vi "interlock v1.vi"() -> ()   [LabVIEW 2015]
panel:
  out "Turbo Status Array":bool[](array[boolean])
  in  "Task to Check Array":refnum<k21>[](array[refnum])
  in  "Test Array":dbl[](array[numeric])
  in  "Turbo Test Array":bool[](array[boolean])
  in  "Manual Test Array":bool[](array[boolean])
  in  "120V Test Array":bool[](array[boolean])
  in  "GV Test Array":bool[](array[boolean])
  out "Manual Control Array":bool[](array[boolean])
  out "120V Relay Signals":refnum<k21>[](array[refnum])
  out "P2L0 in Array":refnum<k21>[](array[refnum])
  out "previous state":bool[](array[boolean])
  out "current state array":bool[](array[boolean])
  out "gv open array":bool[](array[boolean])
  out "gv close array":bool[](array[boolean])
  out "is safe array":bool[](array[boolean])
  out "P0L0 out Array":refnum<k21>[](array[refnum])
  out "P0L16 out Array":refnum<k21>[](array[refnum])
  out "P0L8 in Array":refnum<k21>[](array[refnum])
  in  "Tab Control":enum32{"Page 1"}(tab)
  out "element 5":bool
  out "element 4":bool
  out "Error Indicator":bool
  out "Turbo 1 Status":bool
  out "Turbo 2 Status":bool
  in  "Warnings Cluster":T1
  in  "Turbo Test 1":bool
  in  "Turbo Test 2":bool
  in  "Turbo Test 3":bool
  in  "OK Button":bool
  out "ERROR A":errorcluster
  in  "Beamline 2 Test":dbl
  in  "Beamline 3 Test":dbl
  in  "LEIL Test":dbl
  in  "Turbo 1 Test":dbl
  in  "Turbo 2 Test":dbl
  in  "Turbo 3 Test":dbl
  in  "Post Leil Test":dbl
  in  "Micro Ion Test":dbl
  in  "Beamline 1 Test":dbl
  in  "120V Relay Test 1":bool
  in  "120V Relay Test  2":bool
  in  "120V Relay Test  3":bool
  in  "120V Relay Test  4":bool
  in  "120V Relay Test  5":bool
  in  "120V Relay Test  6":bool
  in  "120V Relay Test  7":bool
  in  "120V Relay Test  8":bool
  in  "Manual Test 1":bool
  in  "Manual Test 2":bool
  in  "Manual Test 3":bool
  in  "Manual Test 4":bool
  in  "Manual Test 5":bool
  in  "Manual Test 6":bool
  in  "Manual Test 7":bool
  in  "Manual Test 8":bool
  in  "GV TEST 1":bool
  in  "GV TEST 2":bool
  in  "GV TEST 3":bool
  in  "GV TEST 4":bool
  in  "GV TEST 5":bool
  in  "GV TEST 6":bool
  in  "GV TEST 7":bool
  in  "GV TEST 8":bool
  in  "TEST MODE":bool
  in  "Pressure Trest Mode":bool
  in  "GV Test Mode":bool
  in  "120 V Status Test Mode":bool
  in  "Turbo Status Test Mode":bool
  in  "Manual Test Mode":bool
  out "SV 1":bool
  out "SV2":bool
  out "SV3":bool
  in  "stop":bool
  out "High Voltage Status":bool
  out "Turbo 2":dbl format="%#_2e"
  in  "OK Button 9":bool
  in  "OK Button 8":bool
  in  "OK Button 7":bool
  in  "OK Button 6":bool
  in  "OK Button 5":bool
  in  "OK Button 4":bool
  in  "OK Button 3":bool
  in  "OK Button 2":bool
  out "GV 8 Status":bool
  out "Gv 7 Status":bool
  out "GV 6 Status":bool
  out "GV 5 Status":bool
  out "GV 4 Status":bool
  out "GV 2 Status":bool
  out "Turbo 2 Backing":bool
  out "Mode 1":bool
  out "Mode 2":bool
  out "Mode 3":bool
  out "Mode 4":bool
  out "Mode 5":bool
  out "GV 1 Status":bool
  out "GV 2 Status":bool
  out "GV 3 Status":bool
  out "GV 4 Status":bool
  out "GV 5 Status":bool
  in  "GV 1":bool
  in  "GV 2":bool
  in  "GV 3":bool
  in  "GV 4":bool
  in  "GV 5":bool
  out "Mode 6":bool
  in  "GV 6":bool
  out "GV 6 Status":bool
  out "Mode 7":bool
  in  "GV 7":bool
  out "GV 7 Status":bool
  out "Mode 8":bool
  in  "GV 8":bool
  out "GV 8 Status":bool
  out "120 V 4 Status":bool
  out "120 V 3 Status":bool
  out "120 V 2 Status":bool
  out "GV 3 Status":bool
  out "GV 1 Status":bool
  out "Cryo 2 Pressure":bool
  out "Cryo 2 Status":bool
  out "Turbo 3 Status":bool
  out "RGA 2 Status":bool
  out "RGA 1 Status":bool
  out "Cryo 1 Status":bool
  out "Cryo 1 Pressure":bool
  out "Beamline 2":dbl format="%#_2e"
  out "Source Electronics Status":bool
  out "Beamline 3":dbl format="%#_2e"
  out "Turbo 1":dbl format="%#_2e"
  out "120 V 1 Status":bool
  out "Micro Ion":dbl format="%#_2e"
  out "Beamline 1":dbl format="%#_2e"
  out "LEIL":dbl format="%#_2e"
  out "Turbo 3":dbl format="%#_2e"
  out "Pos Leil":dbl format="%#_2e"
  out "Post LEIL Pressure":bool
  out "Cryo 2":bool
  out "Beamline 3":bool
  out "Beamline 2 S":bool
  out "LEIL Pressure":bool
  out "Beamline 1 S":bool
  out "Cryo 1":bool
  out "Turbo 1 Backing":bool
  out "Turbo 3 Backing":bool
  out "element":bool
  out "element 2":bool
  out "element 3":bool
  # "RGA 2"
  # "Stutus"
  # "Turbo 1"
  # "Turbo 2"
  # "RGA 1"
  # "Spinning \nStatus"
  # "Turbo 3"
  # "Spinning \nStatus"
  # "Stutus"
  # "Spinning \nStatus"
  # "1\n            2\n            3 \n           4 \n           5  \n          6 \n           7  \n          8"
  # "GV 7"
  # "GV 4"
  # "GV 1"
  # "GV 6"
  # "GV 2"
  # "GV 8"
  # "GV 5"
  # "PSU"
  # "GV 3"
  # "8              7             6             5              4              3              2              1"
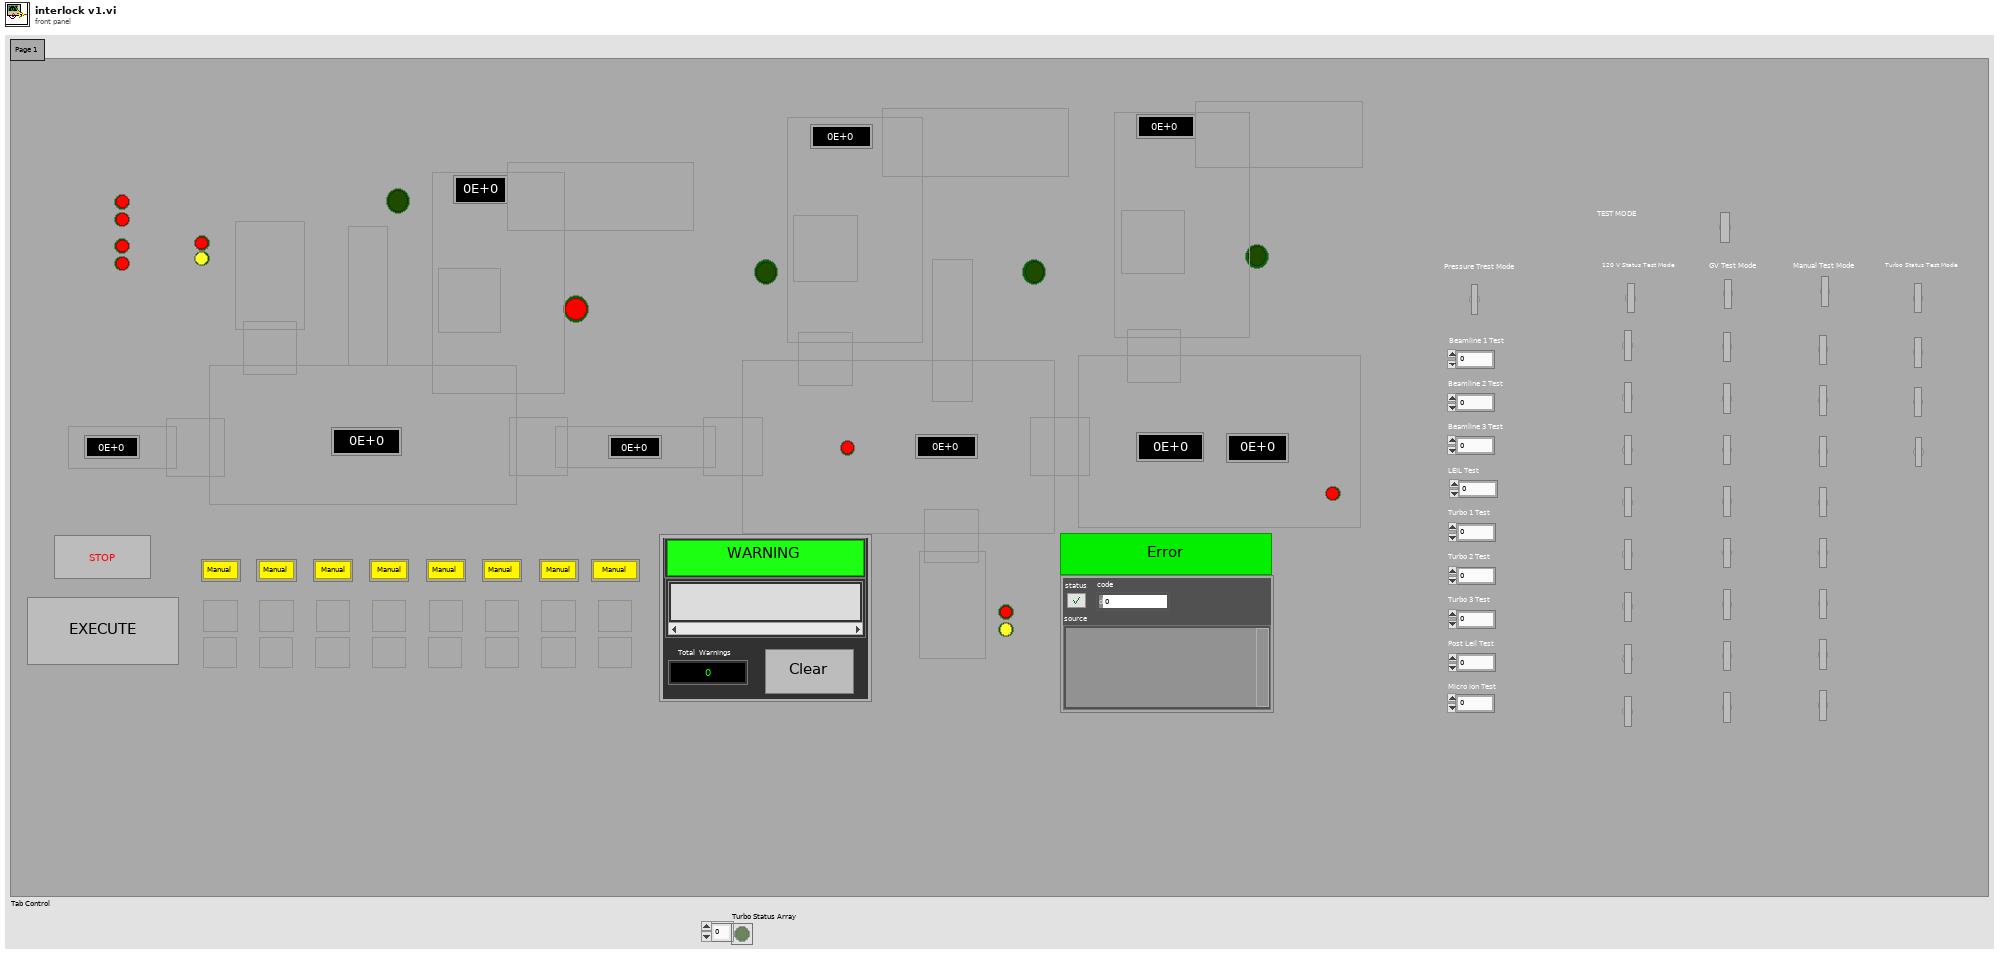
[diagram p1: front panel]
types:
  T1 = cluster{"Warning Array Out":string[], "Clear":bool, "Existing Warnings":i32[], "Num Warning Queue":i32[], "Total  Warnings":i32, "OK Button":bool, "Warning Indicator":bool}
  T2 = enum8{"Enabled", "Disabled", "Disabled and Grayed Out"}
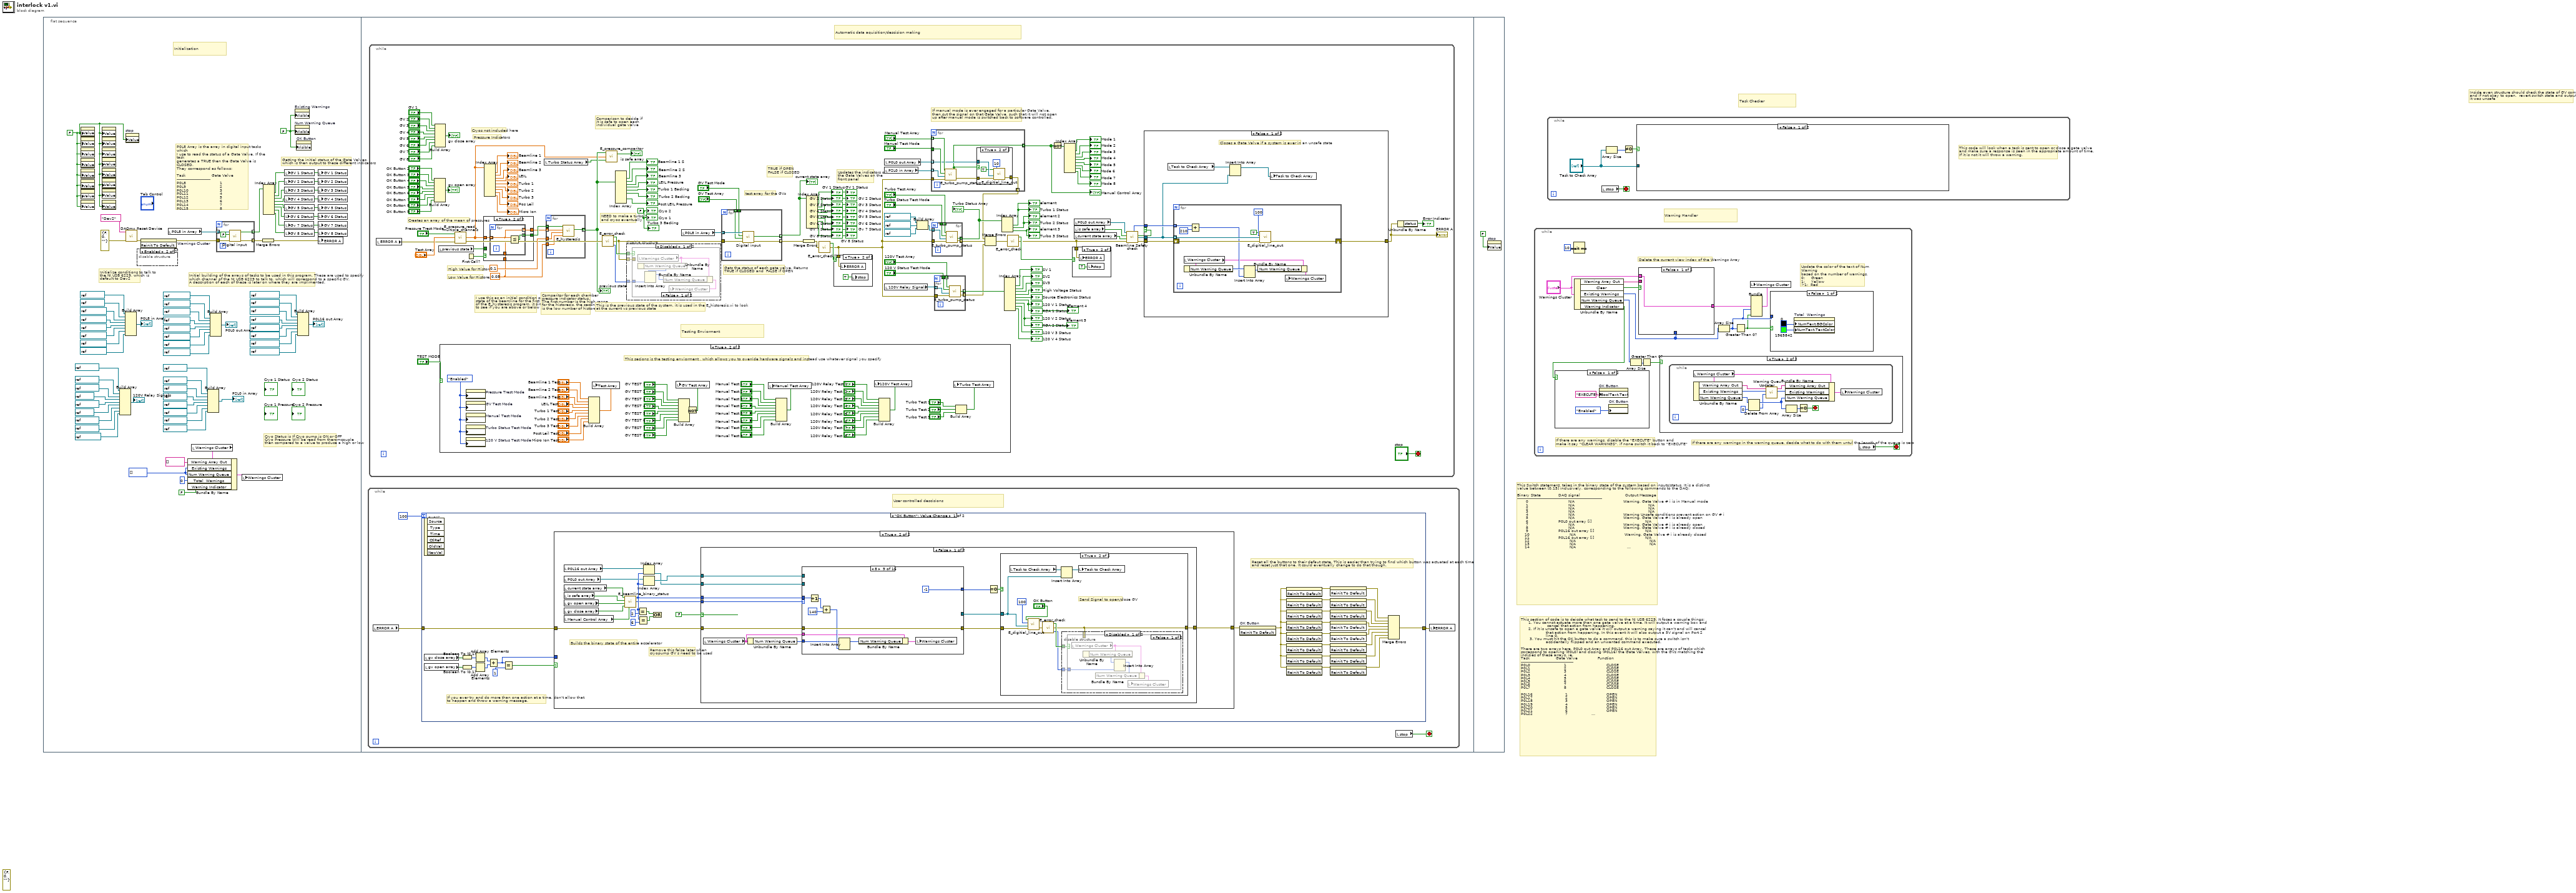
[diagram p0: block diagram]
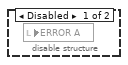
[diagram p2: hidden frame]
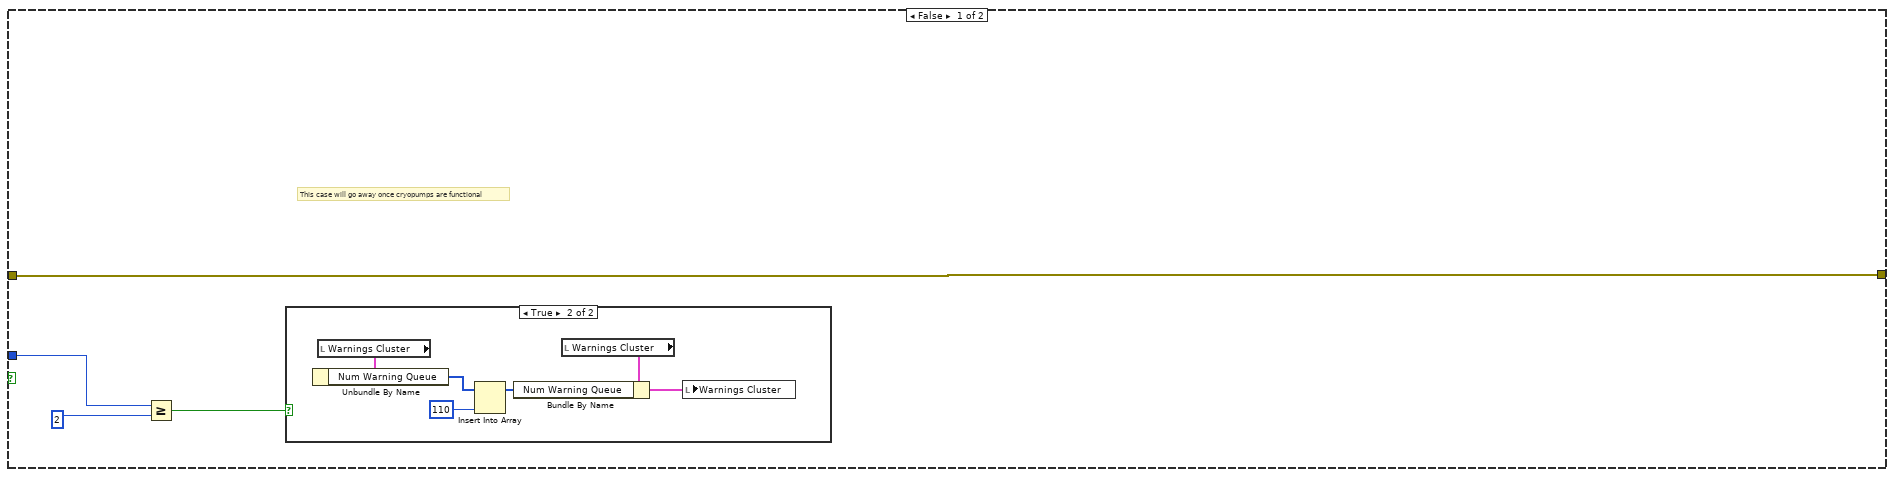
[diagram p3: hidden frame]
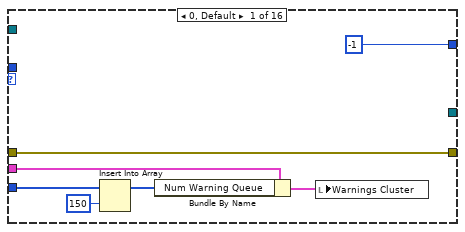
[diagram p5: hidden frame]
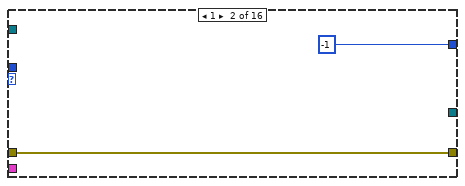
[diagram p6: hidden frame]
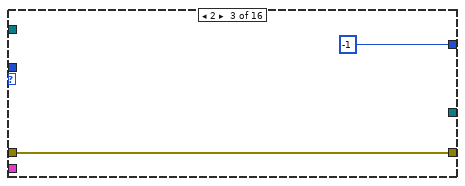
[diagram p7: hidden frame]
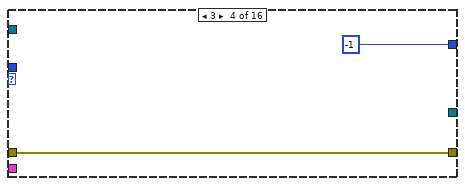
[diagram p8: hidden frame]
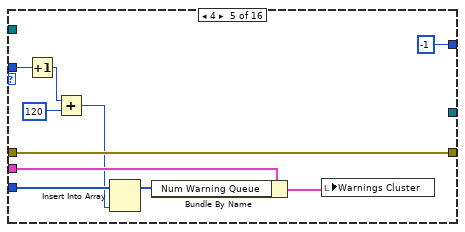
[diagram p9: hidden frame]
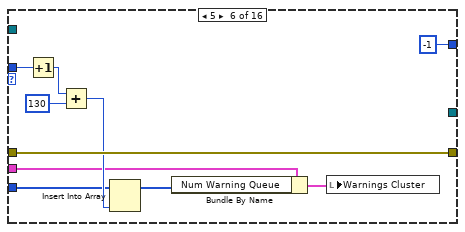
[diagram p10: hidden frame]
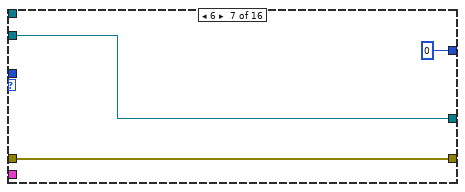
[diagram p11: hidden frame]
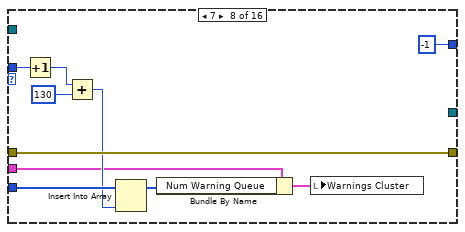
[diagram p12: hidden frame]
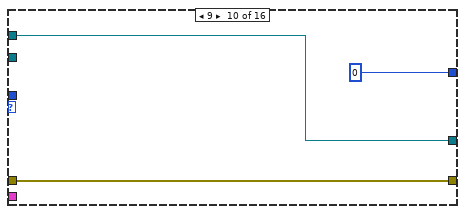
[diagram p13: hidden frame]
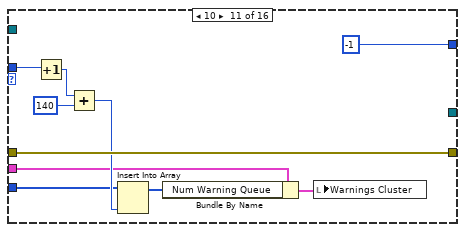
[diagram p14: hidden frame]
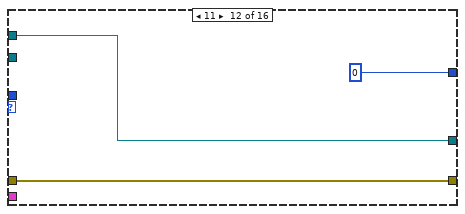
[diagram p15: hidden frame]
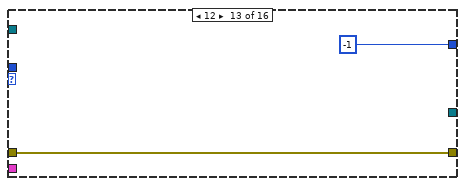
[diagram p16: hidden frame]
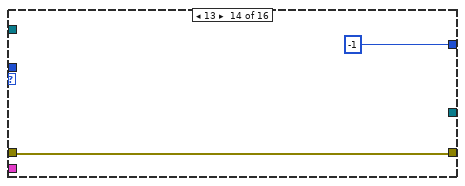
[diagram p17: hidden frame]
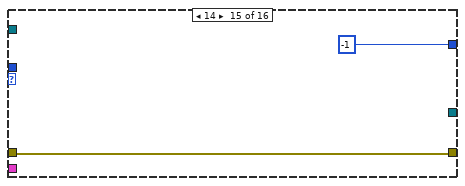
[diagram p18: hidden frame]
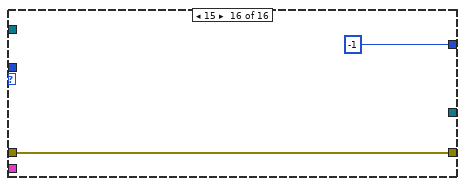
[diagram p19: hidden frame]
diagram:
  (unwired) errorcluster {"status"=FALSE, "code"=0, "source"=""} ("error out")
  # "Task Checker"
  # "Warning Handler"
  # "This Switch statement  takes in the binary state of the system based on inputs/status. It is a distinct\nvalue between [0,15] inclusively, corresponding to the following commands to the DAQ:\n\nBinary State              DAQ signal                                    Output Message\n--------------------------------------------------------------------  \n       0                                N/A                                       Warning, Gate Valve # i is in Manual mode\n       1                                N/A                                                           N/A\n       2                                N/A                                                           N/A\n       3                                N/A                                                           N/A\n       4                                N/A                                       Warning Unsafe conditions prevent action on GV # i\n       5                                N/A                                       Warning, Gate Valve # i is already open\n       6                        P0L0 out array [i]                                           N/A\n       7                                N/A                                       Warning, Gate Valve # i is already open\n       8                                N/A                                       Warning, Gate Valve # i is already closed\n       9                        P0L16 out array [i]                                         N/A\n      10                                N/A                                       Warning, Gate Valve # i is already closed\n      11                       P0L16 out array [i]                                         N/A\n      12                                N/A                                                           N/A\n      13                                N/A                                                           N/A\n      14                                N/A                                                           N/A\n      15                                N/A                                                           N/A\n\nwhere i is the index of the array which corresponds to the Gate valve number.  A description of \nwhat each of these signals does can be found above. \n\nAs a note, the states of between [1,3] inclusively and [12,15] are disallowed states based on the\narchitecture of how the numbers are built and constraints on not being able to have 0 or more than \n1 button hit at a time. I'll consider removing these from the switch statement."
  # "This section of code is to deicde what task to send to the NI USB 6229. It foces a couple things:\n      1. You cannot actuate more than one gate valve at a time. It will output a warning box and \n                     cancel that action from happening.\n      2. If it is unsafe to open a gate valve it will output a warning saying it can't and will cancel \n                    that action from happening. In this event it will also output a 5V signal on Port 2 \n                    line 0.\n       3. You must hit the OK button to do a command, this is to make sure a switch isn't\n                    accidentally flipped and an unwanted command executed.\n\nThere are two arrays here, P0L0 out Array and P0L16 out Array. These are arrays of tasks which \ncorrespond to opening (P0L0) and closing (P0L16) the Gate Valves, with the GVs matching the \nindicies of these arrays. ie. \nTask                     Gate Valve                Function\n------------------------------------------\nP0L0                           1                                CLOSE\nP0L1                           2                                CLOSE\nP0L2                           3                                CLOSE\nP0L3                           4                                CLOSE\nP0L4                           5                                CLOSE\nP0L5                           6                                CLOSE\nP0L6                           7                                CLOSE\nP0L7                           8                                CLOSE\n  \nP0L16                          1                               OPEN\nP0L17                          2                               OPEN\nP0L18                          3                               OPEN\nP0L19                          4                               OPEN\nP0L20                          5                               OPEN\nP0L21                          6                               OPEN\nP0L22                          7                               OPEN\nP0L23                          8                               OPEN"
  # "Inside even structure should check the state of GV comparison array,\nand if not okay to open,  revert switch state and output a message saying\nit was unsafe"
  n1 = flat-sequence {
    frame #0 {
      w2 = FALSE ("GV 1")
      w9 = i32[] [] ("Existing Warnings")
      w13 = FALSE ("Visible")
      # "Initialization"
      # "Cryo Status is If Cryo pump is ON or OFF\nCryo Pressure Will be read from theromcouple \nthen compared to a value to produce a high or low"
      # "Initialize conditions to talk to\nthe NI USB 6229, which is \ndefault to Dev2"
      # "P0L8 Array is the array in digital input tasks which \nI use to read the status of a Gate Valve. If the task\ngenerates a TRUE then the Gate Valve is CLOSED.\nThey corrrespond as follows:\n\nTask                     Gate Valve     \n---------------------------\nP0L8                           1                                \nP0L9                           2                                \nP0L10                         3                               \nP0L11                         4                                \nP0L12                         5                                \nP0L13                         6                                \nP0L14                         7                               \nP0L15                         8"
      # "Getting the initial status of the Gate Valves,\nwhich is then output to these different indicators"
      # "Initial building of the arrays of tasks to be used in this program. These are used to specify\nwhich channel of the NI USB 6229 to talk to, which will correspond to a specific GV. \nA description of each of these is later on where they are implimented."
      n2 = property on="GV 1" class="Bool (strict)"("Value"=w2) -> ()  [unwired: 2 in, 2 out]
      n3 = property on="GV 2" class="Bool (strict)"("Value"=w2) -> ()  [unwired: 2 in, 2 out]
      n4 = property on="GV 3" class="Bool (strict)"("Value"=w2) -> ()  [unwired: 2 in, 2 out]
      n5 = property on="GV 4" class="Bool (strict)"("Value"=w2) -> ()  [unwired: 2 in, 2 out]
      n6 = property on="GV 5" class="Bool (strict)"("Value"=w2) -> ()  [unwired: 2 in, 2 out]
      n7 = property on="GV 6" class="Bool (strict)"("Value"=w2) -> ()  [unwired: 2 in, 2 out]
      n8 = property on="GV 7" class="Bool (strict)"("Value"=w2) -> ()  [unwired: 2 in, 2 out]
      n9 = property on="GV 8" class="Bool (strict)"("Value"=w2) -> ()  [unwired: 2 in, 2 out]
      n10 = property on="OK Button 2" class="Bool (strict)"("Value"=w2) -> ()  [unwired: 2 in, 2 out]
      n11 = property on="OK Button 3" class="Bool (strict)"("Value"=w2) -> ()  [unwired: 2 in, 2 out]
      n12 = property on="OK Button 4" class="Bool (strict)"("Value"=w2) -> ()  [unwired: 2 in, 2 out]
      n13 = property on="OK Button 5" class="Bool (strict)"("Value"=w2) -> ()  [unwired: 2 in, 2 out]
      n14 = property on="OK Button 6" class="Bool (strict)"("Value"=w2) -> ()  [unwired: 2 in, 2 out]
      n15 = property on="OK Button 7" class="Bool (strict)"("Value"=w2) -> ()  [unwired: 2 in, 2 out]
      n16 = property on="OK Button 8" class="Bool (strict)"("Value"=w2) -> ()  [unwired: 2 in, 2 out]
      n17 = property on="OK Button 9" class="Bool (strict)"("Value"=w2) -> ()  [unwired: 2 in, 2 out]
      n18 = Build Array(refnum<k21> "P2L0 in" ("task/channels in"), refnum<k21> "P2L1 in" ("task/channels in"), refnum<k21> "P2L2 in" ("task/channels in"), refnum<k21> "P2L3" ("task/channels in"), refnum<k21> "P2L4 in" ("task/channels in"), refnum<k21> "P2L5" ("task/channels in"), refnum<k21> "P2L6 in" ("task/channels in"), refnum<k21> "P2L7 in" ("element"), refnum<k21> "P0L24 in" ("element")) -> (→"120V Relay Signals":refnum<k21>[])
      n19 = Build Array(refnum<k21> "P0L8 in" ("task/channels in"), refnum<k21> "P0L9 in" ("task/channels in"), refnum<k21> "P0L10 in" ("task/channels in"), refnum<k21> "P0L11 in" ("task/channels in"), refnum<k21> "P0L12 in" ("task/channels in"), refnum<k21> "P0L13 in" ("task/channels in"), refnum<k21> "P0L14 in" ("task/channels in"), refnum<k21> "P0L15 in" ("element")) -> (→"P0L8 in Array":refnum<k21>[])
      n20 = property on="stop" class="Bool (strict)"("Value"=w2) -> ()  [unwired: 2 in, 2 out]
      n21 = call <vilib>:"DAQmx Reset Device.vi"("device in"=tag "Dev2", "error in"=errorcluster {"status"=FALSE, "code"=0, "source"=""} ("error out")) -> ("error out"=w11:errorcluster)  [unwired: 13 in]
      n22 = disable-structure shown="Enabled" {
        frame Disabled {
          n23 = local read "ERROR A"() -> ()  [unwired: 1 in]
        }
        frame Enabled {
        }
      }
      n24 = invoke on="Warnings Cluster" class="Clust (strict)" method="Reinit To Default"(error in=w11) -> (error out=w12:errorcluster)  [unwired: 2 in, 2 out]
      n25 = local read "P0L8 in Array"() -> (w51:refnum<k21>[])
      n26 = local read "Warnings Cluster"() -> (w10:T1)
      n27 = Bundle By Name(cluster=w10, "Warning Array Out"=string[] [], "Existing Warnings"=w9, "Num Warning Queue"=w9, "Total  Warnings"=0, "Warning Indicator"=FALSE) -> (w5:T1)
      n28 = Build Array(refnum<k21> "P1L0 in" ("task/channels in"), refnum<k21> "P1L1 in" ("task/channels in"), refnum<k21> "P1L2 in" ("task/channels in"), refnum<k21> "P1L3 in" ("task/channels in"), refnum<k21> "P1L4 in" ("task/channels in"), refnum<k21> "P1L5 in" ("task/channels in"), refnum<k21> "P1L6 in" ("task/channels in"), refnum<k21> "P1L7 in" ("element")) -> (→"P2L0 in Array":refnum<k21>[])
      n29 = Build Array(refnum<k21> "P0L0 out" ("task/channels in"), refnum<k21> "P0L1 out" ("task/channels in"), refnum<k21> "P0L2 out" ("task/channels in"), refnum<k21> "P0L3 out" ("task/channels in"), refnum<k21> "P0L4 out" ("task/channels in"), refnum<k21> "P0L5 out" ("task/channels in"), refnum<k21> "P0L6 out" ("task/channels in"), refnum<k21> "P0L7 out" ("element")) -> (→"P0L0 out Array":refnum<k21>[])
      n30 = for {
        tunnel: w12 -> [w75]
        tunnel: [w74] -> w69 mode=indexing
        tunnel: w51 -> [w73] mode=indexing
        tunnel: [w72] -> w1 mode=indexing
        n31 = call "Digital input.vi"("error in"=w75, "test"=FALSE, "task/channels in"=w73) -> ("error out"=w74:errorcluster, "element 2"=w72:bool)  [unwired: 7 in]
      }
      n32 = local write "Warnings Cluster"(w5) -> ()
      n33 = Merge Errors(w69) -> (w3:errorcluster)
      n34 = Index Array(array=w1) -> (element #1=w68:bool, element #2=w67:bool, element #3=w66:bool, element #4=w65:bool, element #5=w64:bool, element #6=w63:bool, element #7=w62:bool, element #8=w61:bool)  [unwired: 8 in]
      n35 = local write "GV 6 Status"(w63) -> ()
      n36 = local write "GV 1 Status"(w68) -> ()
      n37 = local write "GV 2 Status"(w67) -> ()
      n38 = local write "GV 3 Status"(w66) -> ()
      n39 = local write "GV 4 Status"(w65) -> ()
      n40 = local write "GV 5 Status"(w64) -> ()
      n41 = local write "Gv 7 Status"(w62) -> ()
      n42 = local write "GV 8 Status"(w61) -> ()
      n43 = property on="Existing Warnings" class="Arr (strict)"("Visible"=w13) -> ()  [unwired: 2 in, 2 out]
      n44 = property on="Num Warning Queue" class="Arr (strict)"("Visible"=w13) -> ()  [unwired: 2 in, 2 out]
      n45 = property on="OK Button" class="Bool (strict)"("Visible"=w13) -> ()  [unwired: 2 in, 2 out]
      n46 = Build Array(refnum<k21> "P0L16 out" ("task/channels in"), refnum<k21> "P0L17 out" ("task/channels in"), refnum<k21> "P0L18 out" ("task/channels in"), refnum<k21> "P0L19 out" ("task/channels in"), refnum<k21> "P0L20 out" ("task/channels in"), refnum<k21> "P0L21 out" ("task/channels in"), refnum<k21> "P0L22 out" ("task/channels in"), refnum<k21> "P0L23 out" ("element")) -> (→"P0L16 out Array":refnum<k21>[])
      n47 = local write "GV 1 Status"(w68) -> ()
      n48 = local write "GV 2 Status"(w67) -> ()
      n49 = local write "GV 3 Status"(w66) -> ()
      n50 = local write "GV 4 Status"(w65) -> ()
      n51 = local write "GV 5 Status"(w64) -> ()
      n52 = local write "GV 6 Status"(w63) -> ()
      n53 = local write "GV 7 Status"(w62) -> ()
      n54 = local write "GV 8 Status"(w61) -> ()
      n55 = local write "ERROR A"(w3) -> ()
    }
    frame #1 {
      # "Automatic data aquisition/descision making"
      n56 = while {
        stop <- w79 stop-if-true
        # "User controlled descisions"
        n57 = local read "ERROR A"() -> (w76:errorcluster)
        n58 = event shown="[0] \"OK Button\": Value Change" {
          selector: _ -> [_ _]
          dyn-events: _ -> [_ _]
          timeout: 100 -> [_ _]
          tunnel: [w83 w256] -> w77
          tunnel: w76 -> [w80 w256]
          event "OK Button": Value Change {
            # "Reset all the buttons to their defaut state. This is easier than trying to find which button was actuated at each time\nand reset just that one. It could eventually change to do that though."
            # "If you ever try and do more than one action at a time, don't allow that \nto happen and throw a warning message."
            n59 = event-data() -> ()  [unwired: 1 in, 6 out]
            n60 = local read "gv close array"() -> (w107:bool[])
            n61 = local read "gv open array"() -> (w108:bool[])
            n62 = Boolean To (0,1)(Boolean=w107) -> (0, 1=w105:i16[])
            n63 = Boolean To (0,1)(Boolean=w108) -> (0, 1=w106:i16[])
            n64 = Add Array Elements(numeric array=w105) -> (sum=w103:i16)
            n65 = Add Array Elements(numeric array=w106) -> (sum=w104:i16)
            n66 = Add(x=w103, y=w104) -> (x+y=w100:i16)
            n67 = Equal?(x=w100, y=i16 1) -> (x = y?=w101:bool)
            n68 = case shown="True" w101 {
              tunnel: w100 -> [w110 _]
              tunnel: [w109 w119] -> w82
              tunnel: w80 -> [w109 w120]
              frame False {
                # "This case will go away once cryopumps are functional"
                n69 = Greater Or Equal?(x=w110, y=i16 2) -> (x >= y?=w111:bool)
                n70 = case shown="True" w111 {
                  frame False {
                  }
                  frame True {
                    n71 = local read "Warnings Cluster"() -> (w114:T1)
                    n72 = Unbundle By Name(w114) -> ("Num Warning Queue"=w118:i32[])
                    n73 = Insert Into Array(array=w118, new element=110) -> (w117:i32[])  [unwired: 1 in]
                    n74 = local read "Warnings Cluster"() -> (w113:T1)
                    n75 = Bundle By Name(cluster=w113, "Num Warning Queue"=w117) -> (w116:T1)
                    n76 = local write "Warnings Cluster"(w116) -> ()
                  }
                }
              }
              frame True {
                # "Builds the binary state of the entire accelerator"
                # "Remove this false later when \ncryopump GV s need to be used"
                n77 = local read "P0L16 out Array"() -> (w127:refnum<k21>[])
                n78 = local read "P0L0 out Array"() -> (w126:refnum<k21>[])
                n79 = local read "current state array"() -> (w125:bool[])
                n80 = local read "is safe array"() -> (w124:bool[])
                n81 = local read "gv open array"() -> (w123:bool[])
                n82 = local read "gv close array"() -> (w122:bool[])
                n83 = local read "Manual Control Array"() -> (w121:bool[])
                n84 = call "E_beamline_binary_status.vi"("Current State Array"=w125, "is safe array"=w124, "gv open aray"=w123, "manual mode array"=w121, "gv closed array"=w122) -> ("index"=w130:i32, "binary state"=w129:i16)  [unwired: 2 in]
                n85 = Equal?(x=w130, y=2) -> (x = y?=w136:bool)
                n86 = Equal?(x=w130, y=6) -> (x = y?=w135:bool)
                n87 = Index Array(array=w127, index=w130) -> (element=w131:refnum<k21>)
                n88 = Index Array(array=w126, index=w130) -> (element=w132:refnum<k21>)
                n89 = Or(x=w136, y=w135) -> ()  [unwired: 1 out]
                n90 = case shown="False" FALSE {
                  tunnel: [w148 w255] -> w119
                  tunnel: w120 -> [w147 w255]
                  tunnel: w132 -> [w146 _]
                  tunnel: w131 -> [w145 _]
                  tunnel: w129 -> [w140 _]
                  tunnel: w130 -> [w139 _]
                  frame False {
                    n91 = local read "Warnings Cluster"() -> (w137:T1)
                    n92 = Unbundle By Name(w137) -> ("Num Warning Queue"=w138:i32[])
                    n93 = case shown="8" w140 {
                      tunnel: [_ _ _ _ _ _ w184 _ _ w207 _ w220 _ _ _ _] -> w144
                      tunnel: w146 -> [_ _ _ _ _ _ _ _ _ w207 _ w220 _ _ _ _]
                      tunnel: w145 -> [_ _ _ _ _ _ w184 _ _ _ _ _ _ _ _ _]
                      tunnel: [-1 -1 -1 -1 -1 -1 0 -1 -1 0 -1 0 -1 -1 -1 -1] -> w143
                      tunnel: w139 -> [_ _ _ _ w165 w180 _ w194 w200 _ w212 _ _ _ _ _]
                      tunnel: w147 -> [w154 w156 w158 w160 w170 w179 w182 w192 w203 w205 w216 w218 w221 w223 w225 w227]
                      tunnel: [w154 w156 w158 w160 w170 w179 w182 w192 w203 w205 w216 w218 w221 w223 w225 w227] -> w141
                      tunnel: w138 -> [w153 _ _ _ w169 w175 _ w189 w198 _ w211 _ _ _ _ _]
                      tunnel: w137 -> [w151 _ _ _ w168 w173 _ w187 w197 _ w209 _ _ _ _ _]
                      frame 0, Default {
                        n94 = Insert Into Array(array=w153, new element=150 ("new element/subarray")) -> (w150:i32[])  [unwired: 1 in]
                        n95 = Bundle By Name(cluster=w151, "Num Warning Queue"=w150) -> (w149:T1)
                        n96 = local write "Warnings Cluster"(w149) -> ()
                      }
                      frame 1 {
                      }
                      frame 2 {
                      }
                      frame 3 {
                      }
                      frame 4 {
                        n97 = Increment(x=w165) -> (x+1=w164:i32)
                        n98 = Add(x=w164, y=120 ("new element/subarray")) -> (x+y=w162:i32)
                        n99 = Insert Into Array(array=w169, new element=w162) -> (w167:i32[])  [unwired: 1 in]
                        n100 = Bundle By Name(cluster=w168, "Num Warning Queue"=w167) -> (w166:T1)
                        n101 = local write "Warnings Cluster"(w166) -> ()
                      }
                      frame 5 {
                        n102 = Increment(x=w180) -> (x+1=w178:i32)
                        n103 = Add(x=w178, y=130) -> (x+y=w176:i32)
                        n104 = Insert Into Array(array=w175, new element=w176) -> (w174:i32[])  [unwired: 1 in]
                        n105 = Bundle By Name(cluster=w173, "Num Warning Queue"=w174) -> (w172:T1)
                        n106 = local write "Warnings Cluster"(w172) -> ()
                      }
                      frame 6 {
                      }
                      frame 7 {
                        n107 = Increment(x=w194) -> (x+1=w190:i32)
                        n108 = Add(x=w190, y=130) -> (x+y=w188:i32)
                        n109 = Insert Into Array(array=w189, new element=w188) -> (w186:i32[])  [unwired: 1 in]
                        n110 = Bundle By Name(cluster=w187, "Num Warning Queue"=w186) -> (w185:T1)
                        n111 = local write "Warnings Cluster"(w185) -> ()
                      }
                      frame 8 {
                        n112 = Increment(x=w200) -> (x+1=w202:i32)
                        n113 = Add(x=w202, y=140) -> (x+y=w199:i32)
                        n114 = Insert Into Array(array=w198, new element=w199) -> (w196:i32[])  [unwired: 1 in]
                        n115 = Bundle By Name(cluster=w197, "Num Warning Queue"=w196) -> (w195:T1)
                        n116 = local write "Warnings Cluster"(w195) -> ()
                      }
                      frame 9 {
                      }
                      frame 10 {
                        n117 = Increment(x=w212) -> (x+1=w215:i32)
                        n118 = Add(x=w215, y=140) -> (x+y=w213:i32)
                        n119 = Insert Into Array(array=w211, new element=w213) -> (w210:i32[])  [unwired: 1 in]
                        n120 = Bundle By Name(cluster=w209, "Num Warning Queue"=w210) -> (w208:T1)
                        n121 = local write "Warnings Cluster"(w208) -> ()
                      }
                      frame 11 {
                      }
                      frame 12 {
                      }
                      frame 13 {
                      }
                      frame 14 {
                      }
                      frame 15 {
                      }
                    }
                    n122 = Equal To 0?(x=w143) -> (x = 0?=w142:bool)
                    n123 = case shown="True" w142 {
                      tunnel: w144 -> [_ w238]
                      tunnel: w141 -> [w229 w239]
                      tunnel: [w229 w230] -> w148
                      frame False {
                      }
                      frame True {
                        # "Send Signal to open/close GV"
                        n124 = local read "Task to Check Array"() -> (w235:refnum<k21>[])
                        n125 = call "E_digitial_line_out.vi"("error in"=w239, "task/channels in"=w238, "milliseconds to wait"=u32 100, "Boolean"="OK Button") -> ("error out"=w233:errorcluster)  [unwired: 2 in]
                        n126 = call "E_error_check.vi"("Error in"=w233) -> ("code"=w231:i32, "Error out"=w230:errorcluster, "Fatal Error"=w232:bool)  [unwired: 2 in]
                        n127 = Insert Into Array(array=w235, new element=w238) -> (w234:refnum<k21>[])  [unwired: 1 in]
                        n128 = disable-structure shown="Disabled" {
                          disable-tunnel: w232 -> [w242 _]
                          disable-tunnel: w231 -> [w241 _]
                          disable-tunnel: w230 -> [w240 _]
                          frame Disabled {
                            n129 = case shown="False" w242 {
                              tunnel: w241 -> [w243 _]
                              tunnel: w240 -> [_ w248]
                              frame False {
                                n130 = local read "Warnings Cluster"() -> (w246:T1)
                                n131 = Unbundle By Name(w246) -> ("Num Warning Queue"=w247:i32[])
                                n132 = Insert Into Array(array=w247, new element=w243) -> (w245:i32[])  [unwired: 1 in]
                                n133 = Bundle By Name(cluster=w246, "Num Warning Queue"=w245) -> (w244:T1)
                                n134 = local write "Warnings Cluster"(w244) -> ()
                              }
                              frame True {
                                n135 = local write "ERROR A"(w248) -> ()
                                n136 = local write "stop"(TRUE ("stop")) -> ()
                              }
                            }
                          }
                          frame Enabled {
                          }
                        }
                        n137 = local write "Task to Check Array"(w234) -> ()
                      }
                    }
                  }
                  frame True {
                    (unwired) "Warning, software control of the Gate valves with cryo pumps on one side are temporarily. Actuation of these must be done manually. " ("message")
                    n138 = local read "Warnings Cluster"() -> (w252:T1)
                    n139 = Unbundle By Name(w252) -> ("Num Warning Queue"=w254:i32[])
                    n140 = Insert Into Array(array=w254, new element=160 ("new element/subarray")) -> (w253:i32[])  [unwired: 1 in]
                    n141 = Bundle By Name(cluster=w252, "Num Warning Queue"=w253) -> (w251:T1)
                    n142 = local write "Warnings Cluster"(w251) -> ()
                  }
                }
              }
            }
            n143 = invoke on="OK Button" class="Bool" method="Reinit To Default"(error in=w82) -> (error out=w81:errorcluster)  [unwired: 2 in, 2 out]
            n144 = invoke on="GV 1" class="Bool (strict)" method="Reinit To Default"(error in=w81) -> (error out=w91:errorcluster)  [unwired: 2 in, 2 out]
            n145 = invoke on="GV 2" class="Bool (strict)" method="Reinit To Default"(error in=w81) -> (error out=w90:errorcluster)  [unwired: 2 in, 2 out]
            n146 = invoke on="GV 3" class="Bool (strict)" method="Reinit To Default"(error in=w81) -> (error out=w89:errorcluster)  [unwired: 2 in, 2 out]
            n147 = invoke on="GV 4" class="Bool (strict)" method="Reinit To Default"(error in=w81) -> (error out=w88:errorcluster)  [unwired: 2 in, 2 out]
            n148 = invoke on="GV 5" class="Bool (strict)" method="Reinit To Default"(error in=w81) -> (error out=w87:errorcluster)  [unwired: 2 in, 2 out]
            n149 = invoke on="GV 6" class="Bool (strict)" method="Reinit To Default"(error in=w81) -> (error out=w86:errorcluster)  [unwired: 2 in, 2 out]
            n150 = invoke on="GV 7" class="Bool (strict)" method="Reinit To Default"(error in=w81) -> (error out=w85:errorcluster)  [unwired: 2 in, 2 out]
            n151 = invoke on="GV 8" class="Bool (strict)" method="Reinit To Default"(error in=w81) -> (error out=w84:errorcluster)  [unwired: 2 in, 2 out]
            n152 = invoke on="OK Button 2" class="Bool (strict)" method="Reinit To Default"(error in=w91) -> (error out=w92:errorcluster)  [unwired: 2 in, 2 out]
            n153 = invoke on="OK Button 3" class="Bool (strict)" method="Reinit To Default"(error in=w90) -> (error out=w93:errorcluster)  [unwired: 2 in, 2 out]
            n154 = invoke on="OK Button 4" class="Bool (strict)" method="Reinit To Default"(error in=w89) -> (error out=w94:errorcluster)  [unwired: 2 in, 2 out]
            n155 = invoke on="OK Button 5" class="Bool (strict)" method="Reinit To Default"(error in=w88) -> (error out=w95:errorcluster)  [unwired: 2 in, 2 out]
            n156 = invoke on="OK Button 6" class="Bool (strict)" method="Reinit To Default"(error in=w87) -> (error out=w96:errorcluster)  [unwired: 2 in, 2 out]
            n157 = invoke on="OK Button 7" class="Bool (strict)" method="Reinit To Default"(error in=w86) -> (error out=w97:errorcluster)  [unwired: 2 in, 2 out]
            n158 = invoke on="OK Button 8" class="Bool (strict)" method="Reinit To Default"(error in=w85) -> (error out=w98:errorcluster)  [unwired: 2 in, 2 out]
            n159 = invoke on="OK Button 9" class="Bool (strict)" method="Reinit To Default"(error in=w84) -> (error out=w99:errorcluster)  [unwired: 2 in, 2 out]
            n160 = Merge Errors(w92, w93, w94, w95, w96, w97, w98, w99) -> (w83:errorcluster)
          }
          event Timeout {
            n161 = event-data() -> ()  [unwired: 1 in, 3 out]
          }
        }
        n162 = local read "stop"() -> (w79:bool)
        n163 = local write "ERROR A"(w77) -> ()
      }
      n164 = while {
        stop <- "stop" stop-if-true
        w276 = FALSE ("Cryo 2")
        w313 = 0.05 ("y")
        # "If manual mode is ever engaged for a particular Gate Valve, \nthen cut the signal on that Gate Valve  such that it will not open\nup after manual mode is switched back to software controlled."
        # "Testing Enviorment"
        # "Gets the status of each gate valve. Returns\nTRUE if CLOSED and  FALSE if OPEN"
        # "Low Value for Historesis"
        # "High Value for Historesis"
        # "Updates the indicators of\nthe Gate Valves on the \nfront panel"
        # "TRUE if OPEN\nFALSE if CLOSED"
        # "This is the previous state of the system, it is used in the E_historesis.vi to look \nat the current vs previous state"
        # "Comparison to decide if\nit is safe to open each\nindividual gate valve"
        # "I use this as an initial condition of the \nstate of the beamline for the first iteration\nof the E_hysteresis program, it simply looks\nto see if you are above or below 1mTorr"
        # "test array for the GVs"
        # "Cryos not included here"
        # "NEED to make a turbo 3\nand cryos eventually"
        # "Pressure Indicators"
        # "Comparitor for each chamber\npressure indicator status.\nThe first number is the high range\nfor the historesis, the second one\nis the low number of historesis."
        # "Creates an array of the mean of pressures"
        n165 = local read "ERROR A"() -> (w268:errorcluster)
        n166 = Build Array("OK Button 2", "OK Button 3", "OK Button 4", "OK Button 5", "OK Button 6", "OK Button 7", "OK Button 8", "OK Button 9") -> (→"gv open array":bool[])
        n167 = Build Array("GV 1", "GV 2", "GV 3", "GV 4", "GV 5", "GV 6", "GV 7", "GV 8") -> (→"gv close array":bool[])
        n168 = local read "previous state"() -> (w331:bool[])
        n169 = case shown="True" "TEST MODE" {
          frame False {
            w412 = FALSE ("Pressure Trest Mode")
            w413 = T2."Disabled and Grayed Out" ("Disabled")
            n170 = property on="GV Test Mode" class="Bool (strict)"("DisabledEnum"=w413) -> ()  [unwired: 2 in, 2 out]
            n171 = property on="Pressure Trest Mode" class="Bool (strict)"("DisabledEnum"=w413) -> ()  [unwired: 2 in, 2 out]
            n172 = property on="Manual Test Mode" class="Bool (strict)"("DisabledEnum"=w413) -> ()  [unwired: 2 in, 2 out]
            n173 = property on="Turbo Status Test Mode" class="Bool (strict)"("DisabledEnum"=w413) -> ()  [unwired: 2 in, 2 out]
            n174 = property on="120 V Status Test Mode" class="Bool (strict)"("DisabledEnum"=w413) -> ()  [unwired: 2 in, 2 out]
            n175 = local write "Pressure Trest Mode"(w412) -> ()
            n176 = local write "120 V Status Test Mode"(w412) -> ()
            n177 = local write "Turbo Status Test Mode"(w412) -> ()
            n178 = local write "Manual Test Mode"(w412) -> ()
            n179 = local write "GV Test Mode"(w412) -> ()
          }
          frame True {
            w456 = T2."Enabled" ("Disabled")
            # "This secions is the testing enviorment , which allows you to override hardware signals and instead use whatever signal you specify"
            n180 = property on="Pressure Trest Mode" class="Bool (strict)"("DisabledEnum"=w456) -> ()  [unwired: 2 in, 2 out]
            n181 = property on="GV Test Mode" class="Bool (strict)"("DisabledEnum"=w456) -> ()  [unwired: 2 in, 2 out]
            n182 = property on="Manual Test Mode" class="Bool (strict)"("DisabledEnum"=w456) -> ()  [unwired: 2 in, 2 out]
            n183 = property on="Turbo Status Test Mode" class="Bool (strict)"("DisabledEnum"=w456) -> ()  [unwired: 2 in, 2 out]
            n184 = property on="120 V Status Test Mode" class="Bool (strict)"("DisabledEnum"=w456) -> ()  [unwired: 2 in, 2 out]
            n185 = Build Array("Beamline 1 Test", "Beamline 2 Test", "Beamline 3 Test", "LEIL Test", "Turbo 1 Test", "Turbo 2 Test", "Turbo 3 Test", "Post Leil Test", "Micro Ion Test") -> (w424:dbl[])
            n186 = local write "Test Array"(w424) -> ()
            n187 = Build Array("GV TEST 1", "GV TEST 2", "GV TEST 3", "GV TEST 4", "GV TEST 5", "GV TEST 6", "GV TEST 7", "GV TEST 8") -> (w447:bool[])
            n188 = Not(x=w447) -> (.not. x?=w414:bool[])
            n189 = local write "GV Test Array"(w414) -> ()
            n190 = Build Array("Manual Test 1", "Manual Test 2", "Manual Test 3", "Manual Test 4", "Manual Test 5", "Manual Test 6", "Manual Test 7", "Manual Test 8") -> (w425:bool[])
            n191 = local write "Manual Test Array"(w425) -> ()
            n192 = Build Array("120V Relay Test 1", "120V Relay Test  2", "120V Relay Test  3", "120V Relay Test  4", "120V Relay Test  5", "120V Relay Test  6", "120V Relay Test  7", "120V Relay Test  8") -> (w427:bool[])
            n193 = local write "120V Test Array"(w427) -> ()
            n194 = Build Array("Turbo Test 1", "Turbo Test 2", "Turbo Test 3") -> (w426:bool[])
            n195 = local write "Turbo Test Array"(w426) -> ()
          }
        }
        n196 = call "E_pressure_read_multiple_channels.vi"("error in"=w268, "Test Array"="Test Array", "Test Mode"="Pressure Trest Mode") -> ("error out"=w274:errorcluster, "Scaled Pressures"=w258:dbl[])  [unwired: 1 in]
        n197 = First Call?() -> (First Call?: T/F=w332:bool)
        n198 = case shown="True" w332 {
          tunnel: w258 -> [w483 w488]
          tunnel: [w484 w487] -> w352
          tunnel: w331 -> [w484 _]
          tunnel: [w483 w486] -> w343
          tunnel: w313 -> [_ w485]
          frame False {
          }
          frame True {
            n199 = for {
              tunnel: w488 -> [w490] mode=indexing
              tunnel: [w491] -> w487 mode=indexing
              tunnel: [w490] -> w486 mode=indexing
              tunnel: w485 -> [w489]
              n200 = Less Or Equal?(x=w490, y=w489) -> (x <= y?=w491:bool)
            }
          }
        }
        n201 = Index Array(array=w258) -> (element #1=→"Beamline 1":dbl, element #2=→"Beamline 2":dbl, element #3=→"Beamline 3":dbl, element #4=→"LEIL":dbl, element #5=→"Turbo 1":dbl, element #6=→"Turbo 2":dbl, element #7=→"Turbo 3":dbl, element #8=→"Pos Leil":dbl, element #9=→"Micro Ion":dbl)  [unwired: 9 in]
        n202 = local read "Turbo Status Array"() -> (w257:bool[])
        n203 = for {
          tunnel: w343 -> [w496] mode=indexing
          tunnel: [w495] -> w259 mode=indexing
          tunnel: w352 -> [w494] mode=indexing
          tunnel: 0.1 ("High Comparitor") -> [w493]
          tunnel: w313 -> [w492]
          n204 = call "E_hysteresis.vi"("Low Comparitor"=w492, "High Comparitor"=w493, "Numeric"=w496, "Previous State"=w494) -> ("Output State"=w495:bool)  [unwired: 3 in]
        }
        "previous state" <- w259
        n205 = call "E_error_check.vi"("Error in"=w274) -> ("code"=w264:i32, "Error out"=w272:errorcluster, "Fatal Error"=w273:bool)  [unwired: 2 in]
        n206 = call "E_pressure_comparitor.vi"("Turbo Status Array"=w257, "Pressures"=w258, "Vacuum State"=w259) -> ("output array"=→"is safe array":bool[])  [unwired: 1 in]
        n207 = Index Array(array=w259) -> (element #1=→"Beamline 1 S":bool, element #2=→"Beamline 2 S":bool, element #3=→"Beamline 3":bool, element #4=→"LEIL Pressure":bool, element #5=→"Turbo 1 Backing":bool, element #6=→"Turbo 2 Backing":bool, element #8=→"Post LEIL Pressure":bool)  [unwired: 9 in, 2 out]
        n208 = disable-structure shown="Disabled" {
          disable-tunnel: w273 -> [w381 _]
          disable-tunnel: w272 -> [w380 _]
          disable-tunnel: w264 -> [w379 _]
          frame Disabled {
            n209 = case shown="False" w381 {
              tunnel: w380 -> [_ w388]
              tunnel: w379 -> [w385 _]
              frame False {
                n210 = local read "Warnings Cluster"() -> (w384:T1)
                n211 = Unbundle By Name(w384) -> ("Num Warning Queue"=w386:i32[])
                n212 = Insert Into Array(array=w386, new element=w385) -> (w383:i32[])  [unwired: 1 in]
                n213 = Bundle By Name(cluster=w384, "Num Warning Queue"=w383) -> (w382:T1)
                n214 = local write "Warnings Cluster"(w382) -> ()
              }
              frame True {
                n215 = local write "ERROR A"(w388) -> ()
                n216 = local write "stop"(TRUE) -> ()
              }
            }
          }
          frame Enabled {
          }
        }
        n217 = local read "P0L8 in Array"() -> (w353:refnum<k21>[])
        n218 = for {
          tunnel: w353 -> [w502] mode=indexing
          tunnel: w272 -> [w501]
          tunnel: [w500] -> w376 mode=indexing
          tunnel: [w497] -> w377 mode=indexing
          tunnel: "GV Test Mode" -> [w499]
          tunnel: "GV Test Array" -> [w498] mode=indexing
          n219 = call "Digital input.vi"("error in"=w501, "test input"=w498, "test"=w499, "task/channels in"=w502) -> ("error out"=w500:errorcluster, "element 2"=w497:bool)  [unwired: 6 in]
        }
        "current state array" <- w377
        n220 = Merge Errors(w376) -> (w271:errorcluster)
        n221 = Index Array(array=w377) -> (element #1=→"GV 1 Status" →"GV 1 Status":bool, element #2=→"GV 2 Status" →"GV 2 Status":bool, element #3=→"GV 3 Status" →"GV 3 Status":bool, element #4=→"GV 4 Status" →"GV 4 Status":bool, element #5=→"GV 5 Status" →"GV 5 Status":bool, element #6=→"GV 6 Status" →"GV 6 Status":bool, element #7=→"GV 7 Status" →"Gv 7 Status":bool, element #8=→"GV 8 Status" →"GV 8 Status":bool)  [unwired: 9 in, 1 out]
        n222 = call "E_error_check.vi"("Error in"=w271) -> ("Error out"=w269:errorcluster, "Fatal Error"=w270:bool)  [unwired: 2 in, 1 out]
        n223 = case shown="True" w270 {
          tunnel: w269 -> [_ w392]
          frame False {
          }
          frame True {
            n224 = local write "ERROR A"(w392) -> ()
            n225 = local write "stop"(TRUE ("stop")) -> ()
          }
        }
        n226 = local read "P0L0 out Array"() -> (w279:refnum<k21>[])
        n227 = local read "P2L0 in Array"() -> (w323:refnum<k21>[])
        n228 = local read "120V Relay Signals"() -> (w307:refnum<k21>[])
        n229 = Build Array(refnum<k21> "P0L25 in" ("task/channels in"), refnum<k21> "P0L26 in" ("task/channels in"), refnum<k21> "P0L27 in" ("task/channels in")) -> (w328:refnum<k21>[])
        n230 = for {
          tunnel: w323 -> [w470] mode=indexing
          tunnel: [w463] -> w277 mode=indexing
          tunnel: w269 -> [w469]
          tunnel: "Manual Test Mode" -> [w468]
          tunnel: "Manual Test Array" -> [w467] mode=indexing
          tunnel: w279 -> [w466] mode=indexing
          tunnel: [w464] -> w278 mode=indexing
          n231 = call "E_turbo_pump_status.vi"("error in"=w469, "task/channels in"=w470, "test mode"=w468, "test value"=w467) -> ("error out"=w465:errorcluster, "element"=w463:bool)  [unwired: 1 in]
          n232 = case shown="True" w463 {
            tunnel: w466 -> [_ w476]
            tunnel: w465 -> [w471 w474]
            tunnel: [w471 w472] -> w464
            frame False {
            }
            frame True {
              n233 = call "E_digitial_line_out.vi"("error in"=w474, "task/channels in"=w476, "milliseconds to wait"=u32 10, "Boolean"=TRUE) -> ("error out"=w472:errorcluster)  [unwired: 2 in]
            }
          }
        }
        "Manual Control Array" <- w277
        n234 = for {
          tunnel: w328 -> [w482] mode=indexing
          tunnel: [w481] -> w324 mode=indexing
          tunnel: w269 -> [w480]
          tunnel: [w479] -> w299 mode=indexing
          tunnel: "Turbo Status Test Mode" -> [w478]
          tunnel: "Turbo Test Array" -> [w477] mode=indexing
          n235 = call "E_turbo_pump_status.vi"("error in"=w480, "task/channels in"=w482, "test mode"=w478, "test value"=w477) -> ("error out"=w479:errorcluster, "element"=w481:bool)  [unwired: 1 in]
        }
        "Turbo Status Array" <- w324
        n236 = for {
          tunnel: w307 -> [w462] mode=indexing
          tunnel: [w461] -> w306 mode=indexing
          tunnel: w269 -> [w460]
          tunnel: [w459] -> w300 mode=indexing
          tunnel: "120 V Status Test Mode" -> [w458]
          tunnel: "120V Test Array" -> [w457] mode=indexing
          n237 = call "E_turbo_pump_status.vi"("error in"=w460, "task/channels in"=w462, "test mode"=w458, "test value"=w457) -> ("error out"=w459:errorcluster, "element"=w461:bool)  [unwired: 1 in]
        }
        n238 = Merge Errors(w278, w299, w300) -> (w267:errorcluster)
        n239 = Index Array(array=w324) -> (element #1=→"Turbo 1 Status" →"element":bool, element #2=→"Turbo 2 Status" →"element 2":bool, element #3=→"Turbo 3 Status" →"element 3":bool)  [unwired: 3 in]
        n240 = Index Array(array=w306) -> (element #1=→"SV 1":bool, element #2=→"SV2":bool, element #3=→"SV3":bool, element #4=→"High Voltage Status":bool, element #5=→"Source Electronics Status":bool, element #6=→"RGA 1 Status" →"120 V 1 Status" →"element 4":bool, element #7=→"RGA 2 Status" →"120 V 2 Status" →"element 5":bool, element #8=→"120 V 3 Status":bool, element #9=→"120 V 4 Status":bool)  [unwired: 9 in]
        n241 = call "E_error_check.vi"("Error in"=w267) -> ("Error out"=w265:errorcluster, "Fatal Error"=w266:bool)  [unwired: 2 in, 1 out]
        n242 = Not(x=w277) -> (.not. x?=w312:bool[])
        n243 = Index Array(array=w312) -> (element #1=→"Mode 1":bool, element #2=→"Mode 2":bool, element #3=→"Mode 3":bool, element #4=→"Mode 4":bool, element #5=→"Mode 5":bool, element #6=→"Mode 6":bool, element #7=→"Mode 7":bool, element #8=→"Mode 8":bool)  [unwired: 8 in]
        n244 = case shown="True" w266 {
          tunnel: w265 -> [_ w390]
          frame False {
          }
          frame True {
            n245 = local write "ERROR A"(w390) -> ()
            n246 = local write "stop"(TRUE) -> ()
          }
        }
        n247 = local read "P0L0 out Array"() -> (w284:refnum<k21>[])
        n248 = local read "is safe array"() -> (w285:bool[])
        n249 = local read "current state array"() -> (w286:bool[])
        n250 = call "Beamline Safety check.vi"("error in"=w265, "Current State Array"=w286, "Is Safe Array"=w285, "Task Array"=w284) -> ("error out"=w283:errorcluster, "Task Array"=w282:refnum<k21>[], "Safe conditions"=w281:bool, "Index Array"=w280:i32[])  [unwired: 3 in, 1 out]
        n251 = case shown="False" w281 {
          tunnel: w283 -> [w398 w411]
          tunnel: [w397 w411] -> w275
          tunnel: w282 -> [w394 _]
          tunnel: w280 -> [w396 _]
          frame False {
            # "Closes a Gate Valve if a system is ever in an unsafe state"
            n252 = local read "Task to Check Array"() -> (w395:refnum<k21>[])
            n253 = for {
              shift-right: [w409] -> w397
              shift-left: w398 -> [w410]
              tunnel: w394 -> [w407] mode=indexing
              tunnel: w396 -> [w405] mode=indexing
              n254 = local read "Warnings Cluster"() -> (w401:T1)
              n255 = Unbundle By Name(w401) -> ("Num Warning Queue"=w406:i32[])
              n256 = Add(x=w405, y=210) -> (x+y=w403:i32)
              n257 = Insert Into Array(array=w406, new element=w403) -> (w402:i32[])  [unwired: 1 in]
              n258 = Bundle By Name(cluster=w401, "Num Warning Queue"=w402) -> (w400:T1)
              n259 = call "E_digitial_line_out.vi"("error in"=w410, "task/channels in"=w407, "milliseconds to wait"=u32 100, "Boolean"=TRUE) -> ("error out"=w409:errorcluster)  [unwired: 2 in]
              n260 = local write "Warnings Cluster"(w400) -> ()
            }
            n261 = Insert Into Array(array=w395, new element=w394) -> (w393:refnum<k21>[])  [unwired: 1 in]
            n262 = local write "Task to Check Array"(w393) -> ()
          }
          frame True {
          }
        }
        "ERROR A" <- w275
        n263 = Unbundle By Name(w275) -> ("status"=→"Error Indicator":bool)
        "Cryo 2" <- w276
        "Cryo 1" <- w276
        "Turbo 3 Backing" <- w276
      }
    }
    frame #2 {
      n264 = property on="stop" class="Bool (strict)"("Value"=FALSE ("stop")) -> ()  [unwired: 2 in, 2 out]
    }
  }
  n265 = while {
    stop <- w517 stop-if-true
    # "If there are any warnings in the warning queue, decide what to do with them untul the length of the queue is zero"
    # "If there are any warnings, disable the \"EXECUTE\" button and\nmake it say \"CLEAR WARNINGS\", if none switch it back to \"EXECUTE\""
    # "Update the color of the text of Num Warning\nbased on the number of warnings, \n0:     Green\n1:     Yellow\n>1:  Red"
    # "Delete the current view index of the Warnings Array"
    n266 = Wait (ms)(milliseconds to wait=u32 10) -> ()  [unwired: 1 out]
    n267 = Unbundle By Name("Warnings Cluster") -> ("Warning Array Out"=w514:string[], "Clear"=w511:bool, "Existing Warnings"=w512:i32[], "Num Warning Queue"=w506:i32[], "Warning Indicator"=w505:bool)
    n268 = case shown="False" w505 {
      frame False {
        n269 = property on="OK Button" class="Bool"("BoolText.Text"="EXECUTE" ("Boolean Text.Text")) -> ()  [unwired: 2 in, 2 out]
        n270 = property on="OK Button" class="Bool"("DisabledEnum"=T2."Enabled" ("Disabled")) -> ()  [unwired: 2 in, 2 out]
      }
      frame True {
        n271 = property on="OK Button" class="Bool"("BoolText.Text"="CLEAR WARINGS" ("Boolean Text.Text")) -> ()  [unwired: 2 in, 2 out]
        n272 = property on="OK Button" class="Bool"("DisabledEnum"=T2."Disabled and Grayed Out" ("Disabled")) -> ()  [unwired: 2 in, 2 out]
      }
    }
    n273 = Array Size(array=w506) -> (size(s)=w516:i32)
    n274 = case shown="False" w511 {
      tunnel: "Warnings Cluster" -> [w531 w541]
      tunnel: w514 -> [_ w540]
      tunnel: w512 -> [_ w539]
      tunnel: [w531 w533] -> w510
      frame False {
      }
      frame True {
        n275 = property on="Warning Array Out" class="Arr (strict)"() -> ("Index Values"=w537:u32[])  [unwired: 2 in, 2 out]
        n276 = Index Array(array=w537, index=0) -> (element=w536:u32)
        n277 = Delete From Array(array=w540, index=w536) -> (array with subset deleted=w535:string[])  [unwired: 1 in, 1 out]
        n278 = Delete From Array(array=w539, index=w536) -> (array with subset deleted=w534:i32[])  [unwired: 1 in, 1 out]
        n279 = Bundle(cluster=w541, "Warning Array Out"=w535, "Clear"=FALSE, "Existing Warnings"=w534) -> (w533:T1)  [unwired: 4 in]
      }
    }
    n280 = Greater Than 0?(x=w516) -> (x > 0?=w515:bool)
    n281 = case shown="True" w515 {
      frame False {
      }
      frame True {
        n282 = while {
          stop <- w550 stop-if-true
          n283 = local read "Warnings Cluster"() -> (w553:T1)
          n284 = Unbundle By Name(w553) -> ("Warning Array Out"=w542:string[], "Existing Warnings"=w547:i32[], "Num Warning Queue"=w548:i32[])
          n285 = Delete From Array(array=w548, index=0) -> (deleted portion=w545:i32, array with subset deleted=w546:i32[])  [unwired: 1 in]
          n286 = call "Warning Queu Updater.vi"("Current Warning Num"=w545, "Existing Num Array"=w547, "Warning Array In"=w542) -> ("Updated Existing Array"=w543:i32[], "Warning Array Out"=w544:string[])  [unwired: 6 in]
          n287 = Bundle By Name(cluster=w553, "Warning Array Out"=w544, "Existing Warnings"=w543, "Num Warning Queue"=w546) -> (w552:T1)
          n288 = Array Size(array=w546) -> (size(s)=w551:i32)
          n289 = Equal To 0?(x=w551) -> (x = 0?=w550:bool)
          n290 = local write "Warnings Cluster"(w552) -> ()
        }
      }
    }
    n291 = Array Size(array=w512) -> (size(s)=w509:i32)
    n292 = Greater Than 0?(x=w509) -> (x > 0?=w508:bool)
    n293 = Bundle(cluster=w510, "Total  Warnings"=w509, "Warning Indicator"=w508) -> (w507:T1)  [unwired: 5 in]
    n294 = local write "Warnings Cluster"(w507) -> ()
    n295 = case shown="False" w508 {
      tunnel: w509 -> [_ w526]
      frame False {
        n296 = property on="Total  Warnings" class="DigNum (strict)"("NumText.BGColor"=u32 0, "NumText.TextColor"=u32 1965842) -> ()  [unwired: 2 in, 2 out]
      }
      frame True {
        n297 = Greater?(x=w526, y=1) -> (0:w524:bool)
        n298 = case shown="False" w524 {
          frame False {
            n299 = property on="Total  Warnings" class="DigNum (strict)"("NumText.BGColor"=u32 0, "NumText.TextColor"=u32 16776704) -> ()  [unwired: 2 in, 2 out]
          }
          frame True {
            n300 = property on="Total  Warnings" class="DigNum (strict)"("NumText.BGColor"=u32 0, "NumText.TextColor"=u32 16720896) -> ()  [unwired: 2 in, 2 out]
          }
        }
      }
    }
    n301 = local read "stop"() -> (w517:bool)
  }
  n302 = while {
    stop <- w557 stop-if-true
    # "This code will look when a task is sent to open or close a gate valve\nand make sure a response is seen in the appropriate amount of time.\nIf it is not it will throw a warning."
    n303 = local read "stop"() -> (w557:bool)
    n304 = Array Size(array="Task to Check Array") -> (size(s)=w555:i32)
    n305 = Not Equal To 0?(x=w555) -> (x != 0?=w556:bool)
    n306 = case shown="False" w556 {
      tunnel: "Task to Check Array" -> [_ w562]
      frame False {
      }
      frame True {
        n307 = call "Signal Checker.vi"("Task to Check Array"=w562, "milliseconds to wait"=u32 100) -> ("Warning Num"=w559:i32)  [unwired: 2 in, 1 out]
        n308 = Not Equal To 0?(x=w559) -> (x != 0?=w560:bool)
        n309 = case shown="True" w560 {
          tunnel: w559 -> [_ w569]
          tunnel: [refnum<k21>[] [] ("Task to Check Array") refnum<k21>[] [] ("Task to Check Array")] -> w558
          frame False {
          }
          frame True {
            n310 = local read "Warnings Cluster"() -> (w567:T1)
            n311 = Unbundle By Name(w567) -> ("Num Warning Queue"=w568:i32[])
            n312 = Insert Into Array(array=w568, new element=w569) -> (w566:i32[])  [unwired: 1 in]
            n313 = Bundle By Name(cluster=w567, "Num Warning Queue"=w566) -> (w565:T1)
            n314 = local write "Warnings Cluster"(w565) -> ()
          }
        }
        n315 = local write "Task to Check Array"(w558) -> ()
      }
    }
  }
